vi "FPGA_controller.vi"() -> ()   [LabVIEW 2017]
uses:
  <vilib>/rvi/Emulation/niFpgaGetClockAttributes.vi
  <vilib>/rvi/Emulation/niFpgaSctlEmulationGetInTimedLoop.vi
  <vilib>/rvi/Emulation/niFpgaEmulationReportErrorSimple.vi
  <vilib>/rvi/eio/common/nirviEmuTemplateMethod_errors.vi
  <vilib>/rvi/Emulation/niFpgaCriticalErrorInLSC.vi
  <vilib>/eio/EIONode/EIONode.xnode
panel:
  out "Translated":i16
  out "VALID":bool
  in  "m_first u2":fxp<+/-,64,32>=-0.8999999999068677 format="%#_42g"
  in  "m_first u1":fxp<+/-,64,32>=-0.8999999999068677 format="%#_42g"
  in  "Scale u2":fxp<+/-,64,42>=5.0 format="%#_35g"
  in  "Offset u2":fxp<+/-,64,41>=2.0 format="%#_36g"
  in  "Scale u1":fxp<+/-,64,42>=5.0 format="%#_35g"
  in  "Offset u1":fxp<+/-,64,41>=2.0 format="%#_36g"
  in  "eta u":fxp<+,16,1>=0.29998779296875 format="%#_42g"
  in  "Scale x2":fxp<+/-,32,16>=10.0 format="%#_21g"
  in  "m_first x2":fxp<+/-,49,33> format="%#_26g"
  in  "Offset x2":fxp<+/-,48,32> format="%#_26g"
  in  "Offset x3":fxp<+/-,48,32>=5.0 format="%#_26g"
  in  "m_first x3":fxp<+/-,32,16>=-3.399993896484375 format="%#_21g"
  in  "Scale x3":fxp<+/-,32,16>=10.0 format="%#_21g"
  in  "1/eta x":fxp<+,3,3>=5.0 format="%#_21g"
  in  "m_first x1":fxp<+/-,49,33> format="%#_26g"
  in  "Offset x1":fxp<+/-,48,32> format="%#_26g"
  in  "Scale x1":fxp<+/-,32,16>=10.0 format="%#_21g"
  in  "stop":bool
  # "INPUTS CONVERSION"
  # "STATES CONVERSION"
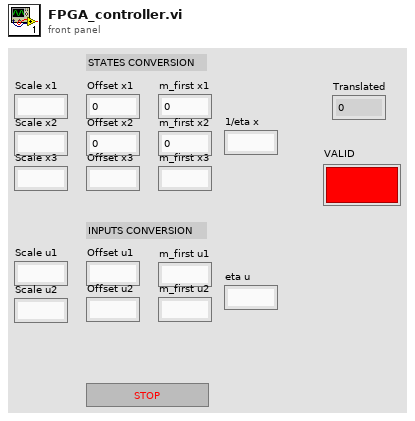
[diagram p1: front panel]
types:
  T1 = cluster{"Boolean array[0]":bool, "Boolean array[1]":bool, "Boolean array[2]":bool, "Boolean array[3]":bool, "Boolean array[4]":bool, "Boolean array[5]":bool, "Boolean array[6]":bool, "Boolean array[7]":bool, "Boolean array[8]":bool, "Boolean array[9]":bool, "Boolean array[10]":bool, "Boolean array[11]":bool, "Boolean array[12]":bool, "Boolean array[13]":bool, "Boolean array[14]":bool, "Boolean array[15]":bool, "Boolean array[16]":bool, "Boolean array[17]":bool}
  T2 = cluster{"Boolean array[0]":bool, "Boolean array[1]":bool, "Boolean array[2]":bool, "Boolean array[3]":bool, "Boolean array[4]":bool, "Boolean array[5]":bool}
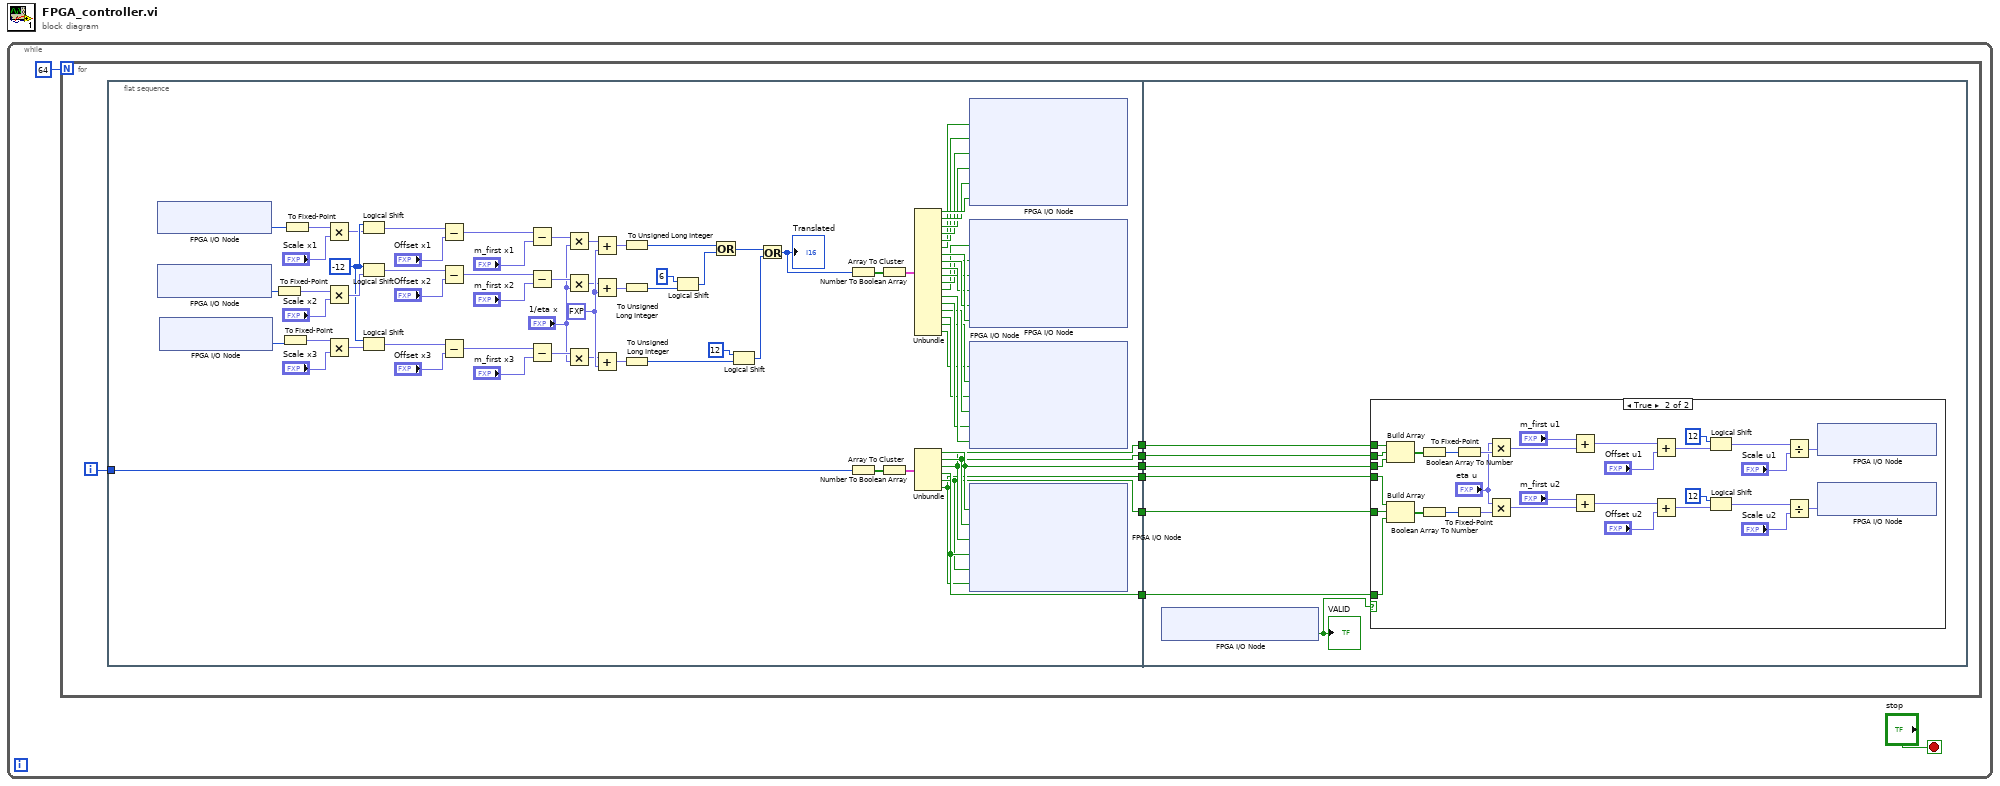
[diagram p0: block diagram]
diagram:
  n1 = while {
    stop <- "stop" stop-if-true
    n2 = for {
      N: 64 -> [_]
      i -> [w9]
      n3 = flat-sequence {
        tunnel: w9 -> [w82]
        tunnel: [w80] -> w8
        tunnel: [w79] -> w7
        tunnel: [w78] -> w6
        tunnel: [w77] -> w5
        tunnel: [w76] -> w4
        tunnel: [w75] -> w3
        tunnel: w8 -> [w90]
        tunnel: w7 -> [w89]
        tunnel: w6 -> [w88]
        tunnel: w5 -> [w87]
        tunnel: w4 -> [w86]
        tunnel: w3 -> [w85]
        frame #0 {
          w44 = fxp<+,2,1> 0.5 ("y")
          w39 = i16 -12 ("y")
          n4 = xnode "FPGA I/O Node"() -> ("ConnectorA/AI0"=w13:u16)  [unwired: 1 in, 1 out]
          n5 = xnode "FPGA I/O Node"() -> ("ConnectorA/AI1"=w15:u16)  [unwired: 1 in, 1 out]
          n6 = xnode "FPGA I/O Node"() -> ("ConnectorB/AI0"=w11:u16)  [unwired: 1 in, 1 out]
          n7 = To Fixed-Point(number=w15) -> (fixed-point=w14:fxp<+,16,16>)  [unwired: 1 in]
          n8 = To Fixed-Point(number=w11) -> (fixed-point=w10:fxp<+,16,16>)  [unwired: 1 in]
          n9 = To Fixed-Point(number=w13) -> (fixed-point=w12:fxp<+,16,16>)  [unwired: 1 in]
          n10 = Multiply(x=w12, y="Scale x1") -> (x*y=w35:fxp<+/-,48,32>)
          n11 = Multiply(x=w14, y="Scale x2") -> (x*y=w45:fxp<+/-,48,32>)
          n12 = Multiply(x=w10, y="Scale x3") -> (x*y=w37:fxp<+/-,48,32>)
          n13 = Logical Shift(y=w39, x=w35) -> (x << y=w32:fxp<+/-,48,32>)
          n14 = Logical Shift(y=w39, x=w45) -> (x << y=w29:fxp<+/-,48,32>)
          n15 = Logical Shift(y=w39, x=w37) -> (x << y=w36:fxp<+/-,48,32>)
          n16 = Subtract(x=w32, y="Offset x1") -> (x-y=w33:fxp<+/-,49,33>)
          n17 = Subtract(x=w29, y="Offset x2") -> (x-y=w30:fxp<+/-,49,33>)
          n18 = Subtract(x=w36, y="Offset x3") -> (x-y=w38:fxp<+/-,49,33>)
          n19 = Subtract(x=w33, y="m_first x1") -> (x-y=w34:fxp<+/-,50,34>)
          n20 = Subtract(x=w30, y="m_first x2") -> (x-y=w28:fxp<+/-,50,34>)
          n21 = Subtract(x=w38, y="m_first x3") -> (x-y=w41:fxp<+/-,50,34>)
          n22 = Multiply(x=w34, y="1/eta x") -> (x*y=w31:fxp<+/-,53,37>)
          n23 = Multiply(x=w28, y="1/eta x") -> (x*y=w27:fxp<+/-,53,37>)
          n24 = Multiply(x=w41, y="1/eta x") -> (x*y=w40:fxp<+/-,52,36>)
          n25 = Add(x=w31, y=w44) -> (x+y=w54:fxp<+/-,53,37>)
          n26 = Add(x=w27, y=w44) -> (x+y=w43:fxp<+/-,53,37>)
          n27 = Add(x=w40, y=w44) -> (x+y=w42:fxp<+/-,52,36>)
          n28 = To Unsigned Long Integer(number=w54) -> (unsigned 32bit integer=w50:u32)
          n29 = To Unsigned Long Integer(number=w43) -> (unsigned 32bit integer=w52:u32)
          n30 = To Unsigned Long Integer(number=w42) -> (unsigned 32bit integer=w48:u32)
          n31 = Logical Shift(y=6, x=w52) -> (x << y=w51:u32)
          n32 = Or(x=w50, y=w51) -> (x .or. y?=w46:u32)
          n33 = Logical Shift(y=12, x=w48) -> (x << y=w47:u32)
          n34 = Or(x=w46, y=w47) -> (x .or. y?=w16:u32)
          "Translated" <- w16
          n35 = Number To Boolean Array(number=w16) -> (Boolean array=w55:bool[])
          n36 = Number To Boolean Array(number=w82) -> (Boolean array=w83:bool[])
          n37 = Array To Cluster(array=w55) -> (cluster=w74:T1)
          n38 = Array To Cluster(array=w83) -> (cluster=w81:T2)
          n39 = Unbundle(w74) -> ("Boolean array[0]"=w73:bool, "Boolean array[1]"=w72:bool, "Boolean array[2]"=w71:bool, "Boolean array[3]"=w70:bool, "Boolean array[4]"=w69:bool, "Boolean array[5]"=w68:bool, "Boolean array[6]"=w67:bool, "Boolean array[7]"=w66:bool, "Boolean array[8]"=w65:bool, "Boolean array[9]"=w64:bool, "Boolean array[10]"=w63:bool, "Boolean array[11]"=w62:bool, "Boolean array[12]"=w61:bool, "Boolean array[13]"=w60:bool, "Boolean array[14]"=w59:bool, "Boolean array[15]"=w58:bool, "Boolean array[16]"=w57:bool, "Boolean array[17]"=w56:bool)
          n40 = Unbundle(w81) -> ("Boolean array[0]"=w80:bool, "Boolean array[1]"=w79:bool, "Boolean array[2]"=w78:bool, "Boolean array[3]"=w77:bool, "Boolean array[4]"=w76:bool, "Boolean array[5]"=w75:bool)
          n41 = xnode "FPGA I/O Node"("Component-Level IP\\pi00"=w68, "Component-Level IP\\pi01"=w69, "Component-Level IP\\pi02"=w70, "Component-Level IP\\pi03"=w71, "Component-Level IP\\pi04"=w72, "Component-Level IP\\pi05"=w73) -> ()  [unwired: 6 in, 6 out]
          n42 = xnode "FPGA I/O Node"("Component-Level IP\\pi06"=w62, "Component-Level IP\\pi07"=w63, "Component-Level IP\\pi08"=w64, "Component-Level IP\\pi09"=w65, "Component-Level IP\\pi10"=w66, "Component-Level IP\\pi11"=w67) -> ()  [unwired: 6 in, 6 out]
          n43 = xnode "FPGA I/O Node"("Component-Level IP\\pi12"=w56, "Component-Level IP\\pi13"=w57, "Component-Level IP\\pi14"=w58, "Component-Level IP\\pi15"=w59, "Component-Level IP\\pi16"=w60, "Component-Level IP\\pi17"=w61) -> ()  [unwired: 6 in, 6 out]
          n44 = xnode "FPGA I/O Node"("Component-Level IP\\pi18"=w80, "Component-Level IP\\pi19"=w79, "Component-Level IP\\pi20"=w78, "Component-Level IP\\pi21"=w77, "Component-Level IP\\pi22"=w76, "Component-Level IP\\pi23"=w75) -> ()  [unwired: 6 in, 6 out]
        }
        frame #1 {
          n45 = xnode "FPGA I/O Node"() -> ("Component-Level IP\\po0"=w84:bool)  [unwired: 1 in, 1 out]
          "VALID" <- w84
          n46 = case shown="True" w84 {
            tunnel: w90 -> [_ w103]
            tunnel: w89 -> [_ w102]
            tunnel: w88 -> [_ w101]
            tunnel: w87 -> [_ w100]
            tunnel: w86 -> [_ w99]
            tunnel: w85 -> [_ w98]
            frame False {
            }
            frame True {
              n47 = Build Array(w101, w102, w103) -> (w120:bool[])
              n48 = Build Array(w98, w99, w100) -> (w111:bool[])
              n49 = Boolean Array To Number(Boolean array=w120) -> (number=w118:u8)
              n50 = Boolean Array To Number(Boolean array=w111) -> (number=w109:u8)
              n51 = To Fixed-Point(number=w118) -> (fixed-point=w117:fxp<+,8,8>)  [unwired: 1 in]
              n52 = To Fixed-Point(number=w109) -> (fixed-point=w108:fxp<+,8,8>)  [unwired: 1 in]
              n53 = Multiply(x="eta u", y=w117) -> (x*y=w121:fxp<+,24,9>)
              n54 = Multiply(x="eta u", y=w108) -> (x*y=w112:fxp<+,24,9>)
              n55 = Add(x="m_first u1", y=w121) -> (x+y=w119:fxp<+/-,64,33>)
              n56 = Add(x="m_first u2", y=w112) -> (x+y=w110:fxp<+/-,64,33>)
              n57 = Add(x=w119, y="Offset u1") -> (x+y=w116:fxp<+/-,64,42>)
              n58 = Add(x=w110, y="Offset u2") -> (x+y=w107:fxp<+/-,64,42>)
              n59 = Logical Shift(y=i16 12, x=w116) -> (x << y=w114:fxp<+/-,64,42>)
              n60 = Logical Shift(y=i16 12, x=w107) -> (x << y=w105:fxp<+/-,64,42>)
              n61 = Divide(x=w114, y="Scale u1") -> (x/y=w113:fxp<+/-,64,65>)
              n62 = Divide(x=w105, y="Scale u2") -> (x/y=w104:fxp<+/-,64,65>)
              n63 = xnode "FPGA I/O Node"("ConnectorB/AO0"=w113) -> ()  [unwired: 1 in, 1 out]
              n64 = xnode "FPGA I/O Node"("ConnectorB/AO1"=w104) -> ()  [unwired: 1 in, 1 out]
            }
          }
        }
      }
    }
  }
